vi "DOReset.vi"(0 "object in":refnum<class "AD2_DO_SDK.lvclass">, 5 "error in (no error)":errorcluster) -> (14 "object out":refnum<class "AD2_DO_SDK.lvclass">, 19 "error out":errorcluster)   [LabVIEW 2021, in "AD2_DO_SDK.lvclass"]
uses:
  AD2_DO_SDK.lvclass
  AD2_DO_SDK.lvclass/AD2_DO_SDK.ctl
  Olasdwf/Olasdwf.lvlib
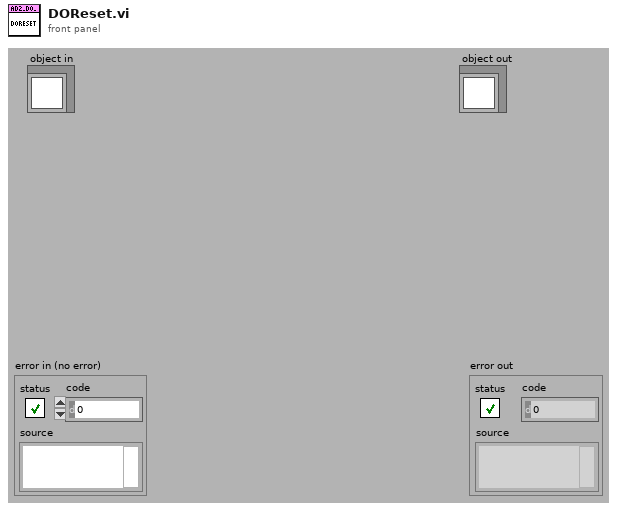
[diagram p1: front panel]
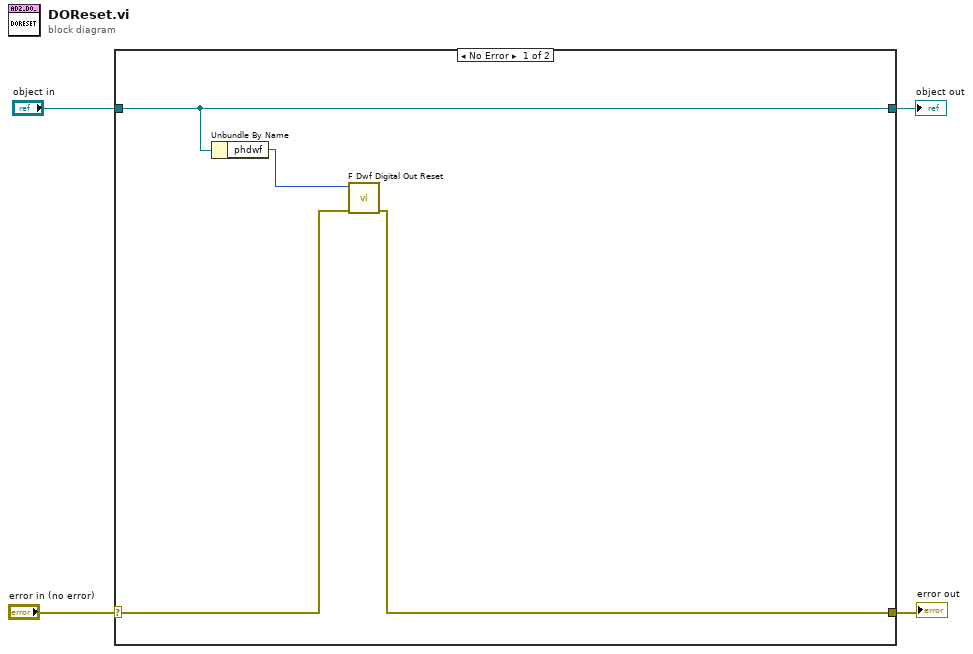
[diagram p0: block diagram]
diagram:
  n1 = case shown="No Error" "error in (no error)" {
    selector: "error in (no error)" -> [w6 w10]
    tunnel: [w5 w10] -> w3
    tunnel: [w8 w9] -> w1
    tunnel: "object in" -> [w8 w9]
    frame No Error {
      n2 = Unbundle By Name(w8) -> ("phdwf"=w7:i32)
      n3 = call "F Dwf Digital Out Reset.vi"("error in (no error)"=w6, "hdwf"=w7) -> ("error out"=w5:errorcluster)  [unwired: 8 in, 1 out]
    }
    frame Error {
    }
  }
  "error out" <- w3
  "object out" <- w1
